vi "PendulumSbrioSide.vi"() -> ()   [LabVIEW 2011]
doc: "This VI was generated automatically using the FPGA Wizard. You can modify the VI normally."
uses:
  <vilib>/Platform/TimedLoop/XDataNode/timing_clust.ctl
  <vilib>/Platform/TimedLoop/XDataNode/nitl_modes.ctl
  <vilib>/Platform/TimedLoop/XDataNode/wakeup.ctl
  <vilib>/FPGAPlugInAG/sbRIO-9632/niLvFpga_Open_sbRIO-9632.vi
  <vilib>/FPGAPlugInAG/sbRIO-9632/niLvFpga_Reset_sbRIO-9632.vi
  <vilib>/FPGAPlugInAG/sbRIO-9632/niLvFpga_Run_sbRIO-9632.vi
  <vilib>/Utility/error.llb/Error Cluster From Error Code.vi
  <vilib>/rvi/errors/niLvFpgaAdjustHostInterfaceError.vi
  <vilib>/FPGAPlugInAG/sbRIO-9632/niLvFpga_Close_sbRIO-9632.vi
  <vilib>/Platform/TimedLoop/XDataNode/XDataNode.xnode
  <vilib>/rvi/interface/nirviOpenFPGA/nirviOpenFPGA.xnode
  FPGA Bitfiles/PPDControlLab3_FPGA_IP5.lvbitx
  <vilib>/rvi/interface/nirviMethod/nirviMethod.xnode
  <vilib>/rvi/interface/nirviReadWriteControl/nirviReadWriteControl.xnode
  <vilib>/rvi/interface/nirviCloseFPGA/nirviCloseFPGA.xnode
  <vilib>/Platform/TimedLoop/XDataNode/XDNodeRunTimeDep.lvlib
  NiFpgaLv.dll
panel:
  in  "Amp Enable":bool
  out "stage difference":i32=11
  out "pendulum difference":i32=1
  in  "pendulum sampling time":u32=10000
  in  "stage sampling time":u32=1000
  out "right limit count":i32=414012
  out "left limit count":i32=-220575
  out "stage position":i32=75902
  out "pendulum angle":i32=110617
  out "error out":errorcluster
  out "Start Acquisition":bool=TRUE
  in  "k4":dbl=-2.5
  in  "k3":dbl=-22.0
  in  "k2":dbl=2.6
  in  "k1":dbl=7.0
  out "Color Box":u32(colorbox)=16711680
  out "stage position (m)":dbl=0.075902
  out "pendulum angle (rad)":dbl=81.7005837531832
  out "stage velocity (m/s)":dbl=0.011
  out "pendulum velocity (rad/s)":dbl=0.07669903939428206
  out "Control Effort":dbl(graph)=-0.05367831515434979
  out "Ref+":fxp<+/-,20,5>=-0.053680419921875 format="%.5g"
  out "Homed":bool=TRUE
  out "Data Ready":bool=TRUE
  out "started":bool=TRUE
  out "right limit":bool
  out "left limit":bool
  in  "Desired Cart Position":dbl(slide) min=-0.220575 max=0.414012 scale=-0.220575..0.414012 scale format="%.4g"
  in  "Local Stop":bool
  in  "Start":bool=TRUE
  in  "Global Stop":bool
  # "Tim, Tim, Raechel & Jon's Gains (Don't Touch)"
  # "ka large\nkb- small\nkc- somewhat big\nkd- somewhat big"
  # "The pendulum velocity was off by an order of magnitude in the previous VI. \nThis mistake has now been corrected in this version."
  # "Team KS\nStep 1 \ninput k1, k2, k3, k4, xmin, xmax\nkp as amplitude of square wave\nkd gain at the limit\nka impulsse"
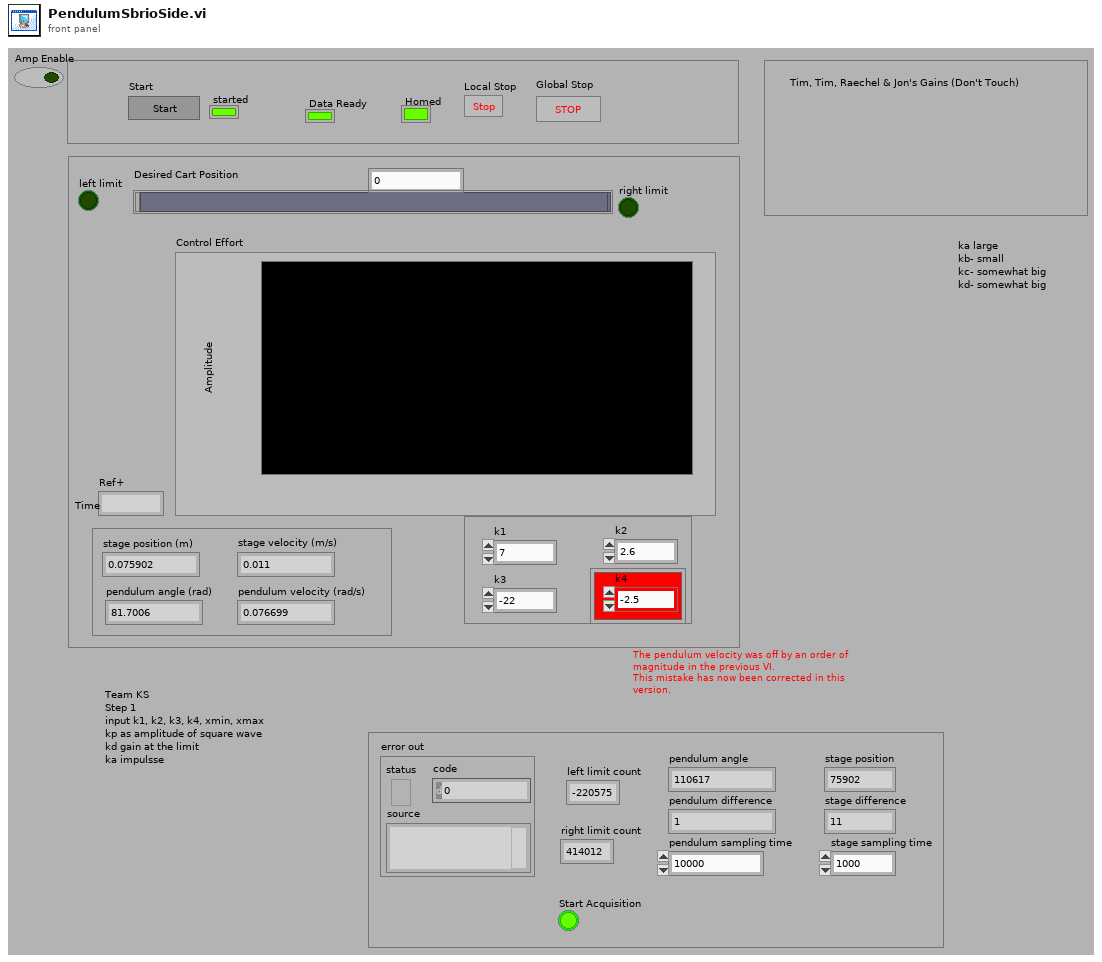
[diagram p1: front panel]
types:
  T1 = cluster{"Angle (cts)":i32, "Angular velocity (cts/s)":dbl, "Position (cts)":i32, "stage velocity (cts/s)":dbl, "time stamp":dbl, "input(v)":dbl}
  T2 = typedef "XDNodeRunTimeDep.lvlib/timing_clust.ctl" = cluster{"Expected End [f-1]":u64, "Actual End [f-1]":u64, "Finished Late? [f-1]":bool, "Expected End [i-1]":u64, "Actual End [i-1]":u64, "Finished Late? [i-1]":bool, "Expected Start [i]":u64, "Actual Start [i]":u64, "Expected Start [f]":u64, "Actual Start [f]":u64, "Source Name":string, "Structure Name":string, "Period":i64, "Deadline":i64, "Offset":i64, "Start":i64, "Priority":i32, "Timeout":i32, "Mode":T3, "Wakeup Reason":T4, "Error":errorcluster, "Source Type":string, "Secondary Source Type":string, "Global End Time":u64, "Global Start Time":u64, "Frame Duration":u64, "Iteration Duration":u64, "Assigned CPU":i32, "I/O Scan Engine Mode":u32}
  T3 = typedef "XDNodeRunTimeDep.lvlib/nitl_modes.ctl" = enum32{"No Change", "Process missed periods, maintain original phase", "Discard missed periods, maintain original phase", "Process missed periods, ignore original phase", "Discard missed periods, ignore original phase"}
  T4 = typedef "XDNodeRunTimeDep.lvlib/wakeup.ctl" = enum32{"Normal", "Aborted", "Asynchronous wakeup", "Timing source error", "Timed loop error", "Timeout"}
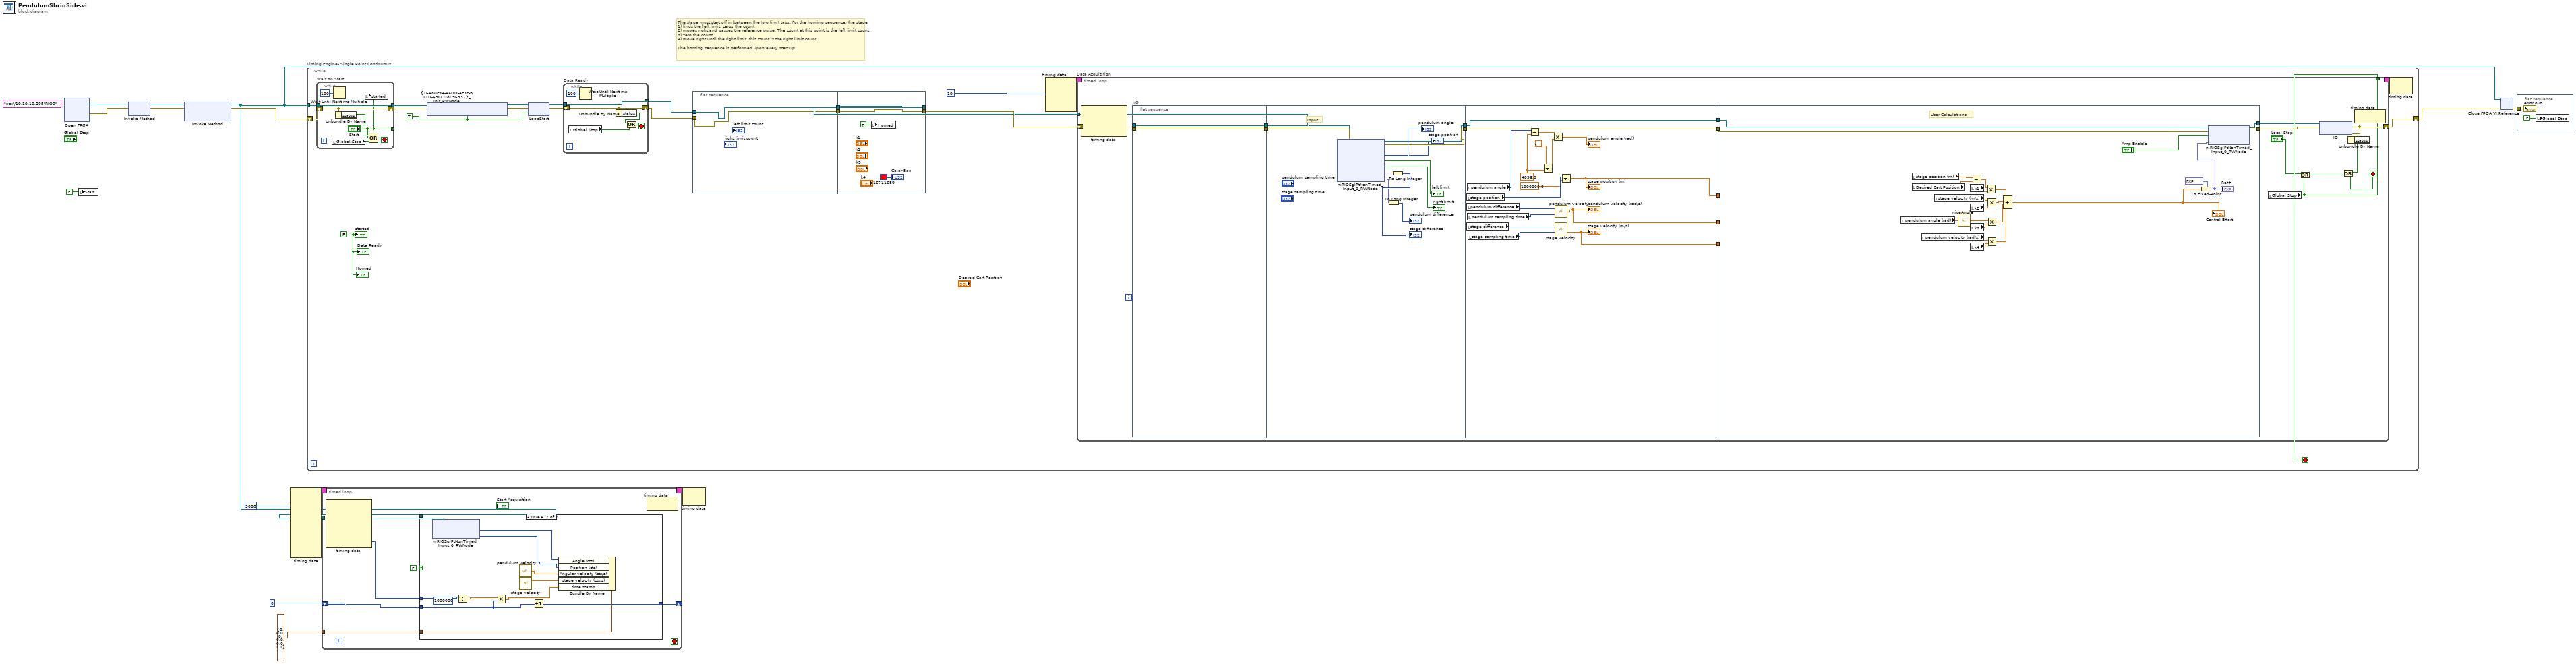
[diagram p0: block diagram]
diagram:
  # "The stage must start off in between the two limit tabs. For the homing sequence, the stage\n1) finds the left limit, zeros the count\n2) moves right and passes the reference pulse. The count at this point is the left limit count\n3) zero the count\n4) move right until the right limit, this count is the right limit count.\n\nThe homing sequence is performed upon every start up."
  n1 = xnode ("Open FPGA")("resource name"=tag "rio://10.10.10.205/RIO0") -> ("FPGA VI Reference Out"=w11:refnum<k20>, "error out"=w12:errorcluster)  [unwired: 1 in]
  n2 = local write "Start"(FALSE ("Start 0")) -> ()
  n3 = xnode ("Invoke Method")("FPGA VI Reference In"=w11, "error in"=w12) -> ("FPGA VI Reference Out"=w14:refnum<k20>, "error out"=w15:errorcluster)
  n4 = xnode ("Invoke Method")("FPGA VI Reference In"=w14, "error in"=w15) -> ("FPGA VI Reference Out"=w3:refnum<k20>, "error out"=w13:errorcluster)  [unwired: 1 in]
  n5 = node-c288(i64 5000 ("Period")) -> (w8:T2)  [unwired: 9 in]
  n6 = while "Timing Engine- Single Point Continuous" {
    tunnel: w3 -> [w35]
    shift-right: [w34] -> w10
    shift-left: w13 -> [w36]
    stop <- w27 stop-if-true
    w21 = FALSE
    w16 = TRUE ("const")
    n7 = while "Wait on Start" {
      tunnel: w35 -> [w133]
      tunnel: [w133] -> w29
      tunnel: ["Start"] -> _
      shift-right: [w130] -> w28
      shift-left: w36 -> [w130]
      stop <- w134 stop-if-true
      n8 = local read "Global Stop"() -> (w131:bool)
      n9 = Wait Until Next ms Multiple(millisecond multiple=u32 100) -> ()  [unwired: 1 out]
      n10 = Unbundle By Name(w130) -> ("status"=w129:bool)
      n11 = local write "started"("Start") -> ()
      n12 = Compound Arithmetic op=OR(w129, "Start", w131) -> (w134:bool)
    }
    n13 = xnode ("{16A80F94-AADD-4F3F-B01D-65CCD8C96937}_Init_RWNode")("FPGA VI Reference In"=w29, "error in"=w28, "quad reset (Port0/DIO0,Port0/DIO1)"=w16) -> ("FPGA VI Reference Out"=w31:refnum<k20>, "error out"=w30:errorcluster)
    n14 = xnode ("LoopStart")("FPGA VI Reference In"=w31, "error in"=w30, "Start 0"=w16) -> ("FPGA VI Reference Out"=w33:refnum<k20>, "error out"=w32:errorcluster)
    n15 = while "Data Ready" {
      tunnel: w33 -> [w123]
      tunnel: [w123] -> w25
      shift-right: [w122] -> w20
      shift-left: w32 -> [w122]
      stop <- w125 stop-if-true
      n16 = local read "Global Stop"() -> (w126:bool)
      n17 = Wait Until Next ms Multiple(millisecond multiple=u32 100) -> ()  [unwired: 1 out]
      n18 = Unbundle By Name(w122) -> ("status"=w124:bool)
      n19 = Compound Arithmetic op=OR(w124, w126) -> (w125:bool)
    }
    n20 = flat-sequence {
      tunnel: w20 -> [w116]
      tunnel: w25 -> [w117]
      tunnel: [w116] -> w23
      tunnel: [w117] -> w22
      tunnel: [w119] -> w24
      tunnel: [w118] -> w26
      tunnel: w23 -> [w118]
      tunnel: w22 -> [w119]
      frame #0 {
      }
      frame #1 {
        n21 = local write "Homed"(TRUE ("Homed")) -> ()
        "Color Box" <- u32 16711680 ("Color Box")
      }
    }
    n22 = node-c288(i64 10 ("Period")) -> (w19:T2)  [unwired: 3 in]
    n23 = timed-loop "Data Acquisition" {
      tunnel: w24 -> [w50]
      tunnel: [w52] -> w27
      shift-right: [w53] -> w34
      shift-left: w26 -> [w49]
      timing: w19 -> [_]
      timing-out: [_] -> w18
      stop <- w47 stop-if-true
      n24 = node-c288() -> ()  [unwired: 1 in, 4 out]
      n25 = flat-sequence "I/O" {
        tunnel: w49 -> [w58]
        tunnel: w50 -> [w59]
        tunnel: [w59] -> w44
        tunnel: [w58] -> w43
        tunnel: [w70] -> w46
        tunnel: [w68] -> w45
        tunnel: w44 -> [w69]
        tunnel: w43 -> [w71]
        tunnel: [w88] -> w42
        tunnel: [w87] -> w41
        tunnel: w45 -> [w87]
        tunnel: w46 -> [w88]
        tunnel: [w74] -> w40
        tunnel: [w73] -> w39
        tunnel: [w72] -> w38
        tunnel: w42 -> [w109]
        tunnel: w41 -> [w111]
        tunnel: [w108] -> w55
        tunnel: [w110] -> w54
        tunnel: w40 -> [_]
        tunnel: w39 -> [_]
        tunnel: w38 -> [_]
        frame #0 {
        }
        frame #1 {
          # "Input"
          n26 = xnode ("niRIOSglPtNonTimed_Input_0_RWNode")("FPGA VI Reference In"=w69, "error in"=w71) -> ("FPGA VI Reference Out"=w68:refnum<k20>, "error out"=w70:errorcluster, "Pendulum Position"=→"pendulum angle":i32, "Stage Position"=→"stage position":i32, "Left Limit"=→"left limit":bool, "Right Limit"=→"right limit":bool, "Delta_X"=w63:fxp<+/-,33,33>, "Delta_theta"=w61:fxp<+/-,33,33>)
          n27 = To Long Integer(number=w61) -> (32bit integer=→"pendulum difference":i32)
          n28 = To Long Integer(number=w63) -> (32bit integer=→"stage difference":i32)
        }
        frame #2 {
          w77 = 4096.0 ("y")
          n29 = local read "stage position"() -> (w80:i32)
          n30 = local read "pendulum difference"() -> (w83:i32)
          n31 = local read "stage difference"() -> (w86:i32)
          n32 = local read "pendulum angle"() -> (w76:i32)
          n33 = local read "pendulum sampling time"() -> (w85:u32)
          n34 = local read "stage sampling time"() -> (w84:u32)
          n35 = Subtract(x=w76, y=w77) -> (x-y=w78:dbl)
          n36 = Divide(x=3.141592653589793, y=w77) -> (x/y=w82:dbl)
          n37 = Multiply(x=w78, y=w82) -> (x*y=→"pendulum angle (rad)":dbl)
          n38 = call "pendulum velocity.vi"("Pendulum Sampling Time"=w85, "Pendulum Count"=w83) -> ("pendulum velocity (rad/s)"=w74:dbl)
          "pendulum velocity (rad/s)" <- w74
          n39 = call "stage velocity.vi"("Stage Sampling Time"=w84, "Stage Count"=w86) -> ("stage velocity (m/s)"=w72:dbl)
          "stage velocity (m/s)" <- w72
          n40 = Divide(x=w80, y=1000000.0) -> (x/y=w73:dbl)
          "stage position (m)" <- w73
        }
        frame #3 {
          # "User Calculations"
          n41 = local read "pendulum angle (rad)"() -> (w92:dbl)
          n42 = local read "stage position (m)"() -> (w96:dbl)
          n43 = local read "Desired Cart Position"() -> (w94:dbl)
          n44 = local read "pendulum velocity (rad/s)"() -> (w102:dbl)
          n45 = local read "stage velocity (m/s)"() -> (w93:dbl)
          n46 = call "niceAngle.vi"("radian"=w92) -> ("radian out"=w91:dbl)
          n47 = local read "k1"() -> (w101:dbl)
          n48 = local read "k2"() -> (w97:dbl)
          n49 = local read "k3"() -> (w104:dbl)
          n50 = local read "k4"() -> (w103:dbl)
          n51 = Subtract(x=w96, y=w94) -> (x-y=w95:dbl)
          n52 = Multiply(x=w95, y=w101) -> (x*y=w100:dbl)
          n53 = Multiply(x=w93, y=w97) -> (x*y=w105:dbl)
          n54 = Multiply(x=w91, y=w104) -> (x*y=w99:dbl)
          n55 = Multiply(x=w102, y=w103) -> (x*y=w98:dbl)
          n56 = Compound Arithmetic op=ADD(w100, w105, w99, w98) -> (w106:dbl)
          "Control Effort" <- w106
          n57 = To Fixed-Point(fixed-point type=fxp<+/-,20,5> 0.0 ("Ref+ 2"), number=w106) -> (fixed-point=w90:fxp<+/-,20,5>)
          "Ref+" <- w90
          n58 = xnode ("niRIOSglPtNonTimed_Input_0_RWNode")("FPGA VI Reference In"=w111, "error in"=w109, "Amp Enable"="Amp Enable", "Amp Cpmmand"=w90) -> ("FPGA VI Reference Out"=w110:refnum<k20>, "error out"=w108:errorcluster)
        }
      }
      n59 = local read "Global Stop"() -> (w52:bool)
      n60 = Or(x="Local Stop", y=w52) -> (x .or. y?=w37:bool)
      n61 = xnode ("IO")("FPGA VI Reference In"=w54, "error in"=w55) -> ("error out"=w53:errorcluster)  [unwired: 1 in, 1 out]
      n62 = Unbundle By Name(w53) -> ("status"=w51:bool)
      n63 = Or(x=w51, y=w37) -> (x .or. y?=w47:bool)
      n64 = node-c288() -> ()  [unwired: 1 in, 1 out]
    }
    n65 = node-c288(w18) -> ()  [unwired: 1 out]
    "started" <- w21
    "Data Ready" <- w21
    "Homed" <- w21
  }
  n66 = timed-loop {
    timing: w8 -> [_]
    timing-out: [_] -> w7
    shift-right: [w139] -> _
    shift-left: 0 -> [w138]
    tunnel: w3 -> [w137]
    tunnel: T1 {"Angle (cts)"=0, "Angular velocity (cts/s)"=0.0, "Position (cts)"=0, "stage velocity (cts/s)"=0.0, "time stamp"=0.0, "input(v)"=0.0} ("output cluster") -> [w136]
    stop <- _ stop-if-true
    n67 = node-c288() -> (w140:i64)  [unwired: 1 in, 6 out]
    n68 = case shown="True" FALSE {
      tunnel: w140 -> [_ w147]
      tunnel: [w141 w153] -> w139
      tunnel: w138 -> [w141 w151]
      tunnel: w137 -> [_ w152]
      tunnel: w136 -> [_ w144]
      frame False {
      }
      frame True {
        n69 = xnode ("niRIOSglPtNonTimed_Input_0_RWNode")("FPGA VI Reference In"=w152) -> ("Pendulum Position"=w143:i32, "Stage Position"=w142:i32)  [unwired: 1 in, 2 out]
        n70 = Divide(x=w147, y=i64 1000000) -> (x/y=w145:dbl)
        n71 = Multiply(x=w145, y=w151) -> (x*y=w150:dbl)
        n72 = call "pendulum velocity.vi"() -> ("pendulum velocity (rad/s)"=w149:dbl)  [unwired: 2 in]
        n73 = call "stage velocity.vi"() -> ("stage velocity (m/s)"=w148:dbl)  [unwired: 2 in]
        n74 = Increment(x=w151) -> (x+1=w153:i32)
        n75 = Bundle By Name(cluster=w144, "Angle (cts)"=w143, "Position (cts)"=w142, "Angular velocity (cts/s)"=w149, "stage velocity (cts/s)"=w148, "time stamp"=w150) -> ()  [unwired: 1 out]
      }
    }
    n76 = node-c288() -> ()  [unwired: 1 in, 1 out]
  }
  n77 = node-c288(w7) -> ()  [unwired: 1 out]
  n78 = xnode ("Close FPGA VI Reference")("FPGA VI Reference In"=w3, "error in"=w10) -> ("error out"=w9:errorcluster)
  n79 = flat-sequence {
    tunnel: w9 -> [w158]
    frame #0 {
      n80 = local write "Global Stop"(FALSE ("Global Stop")) -> ()
      "error out" <- w158
    }
  }
